vi "EventLog.Gui.Stop.vi"(8 "error in":errorcluster, 11 "Ref":refnum<vi>) -> (0 "error out":errorcluster)   [LabVIEW 2016]
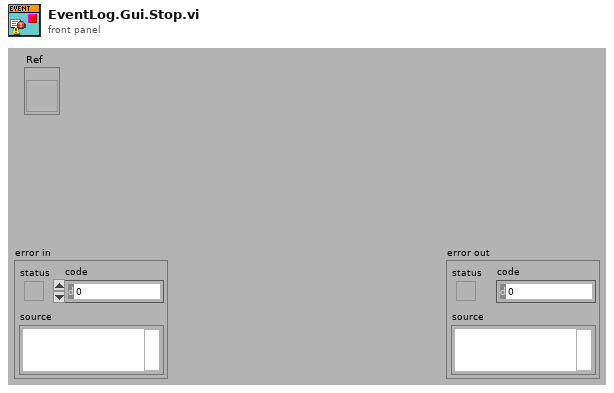
[diagram p1: front panel]
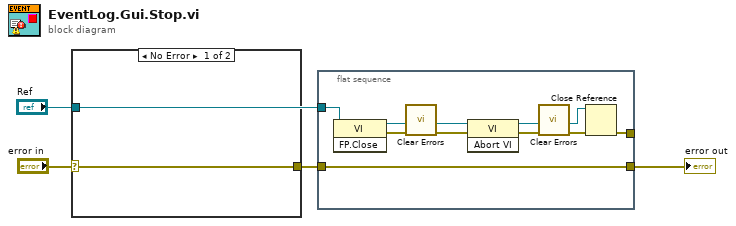
[diagram p0: block diagram]
diagram:
  n1 = case shown="No Error" "error in" {
    selector: "error in" -> [w5 w6]
    tunnel: "Ref" -> [_ _]
    tunnel: [w5 w6] -> w3
    frame No Error {
    }
    frame Error {
    }
  }
  n2 = flat-sequence {
    tunnel: w3 -> [w15]
    tunnel: "Ref" -> [w8]
    tunnel: [w15] -> w1
    tunnel: [w14] -> _
    frame #0 {
      n3 = invoke class="VI" method="FP.Close"(reference=w8) -> (reference out=w12:refnum<vi>, error out=w13:errorcluster)  [unwired: 2 in, 1 out]
      n4 = call <vilib>:"Clear Errors.vi"("error in (no error)"=w13) -> ("error out"=w11:errorcluster)  [unwired: 5 in, 1 out]
      n5 = invoke class="VI" method="Abort VI"(reference=w12, error in=w11) -> (reference out=w7:refnum<vi>, error out=w10:errorcluster)  [unwired: 1 in, 1 out]
      n6 = call <vilib>:"Clear Errors.vi"("error in (no error)"=w10) -> ("error out"=w9:errorcluster)  [unwired: 5 in, 1 out]
      n7 = Close Reference(reference=w7, error in (no error)=w9) -> (error out=w14:errorcluster)
    }
  }
  "error out" <- w1
